vi "Exposure-Brickwall Noise.vi"(1 "seed":i32=-1, 7 "InvFilt Params":T3={"Min Frequency (Hz)"=0.0, "Max Frequency (Hz)"=0.0, "Length (points)"=301, "Sampling rate (Hz)"=0.0, "Delay (ms)"=301.0, "Linear phase"=FALSE}, 9 "Brickwall (T)":bool=TRUE, 11 "error in (no error)":errorcluster) -> (4 "Noise":dbl[](array[numeric]), 8 "dB":dbl[](array[numeric]), 15 "error out":errorcluster)   [LabVIEW 2020]
uses:
  epl-cal-vi-lib/Inverse Filter VIs/InvFilt-Params.ctl
  epl-vi-lib/Signal Synthesis VIs/Controls/Advanced Filter XCtl/Filter Data.ctl
  epl-vi-lib/Signal Synthesis VIs/Filter VIs/Filter-Bandwidth Units.ctl
  epl-vi-lib/Signal Synthesis VIs/Waveform VIs/Noise VIs/Noise-Globals.vi
  epl-vi-lib/Utility VIs/Math VIs/FFT x(t) to dB,Degrees (1D).vi
  epl-vi-lib/Utility VIs/Math VIs/Linear to dB (array).vi
  <vilib>/Analysis/NI_AALBase.lvlib
  epl-vi-lib/Signal Synthesis VIs/Controls/Advanced Filter XCtl/Advanced Filter XCtl.xctl
panel:
  in  "Filter in":T1={"Type"=enum."Bandpass", "CF (kHz)"=0.0, "BW (kHz)"=0.0, "Cascade"=TRUE, "Quadrature"=FALSE, "Scale Factor"=0.0, "Stages"=[], "Class"=enum."Elliptic", "Order"=7, "BWUnits"=enum."Linear"} {"Stages"."IIR Filter"."Forward Coefficients" format="%.4f"; "Stages"."IIR Filter"."Reverse Coefficients" format="%.4f"}
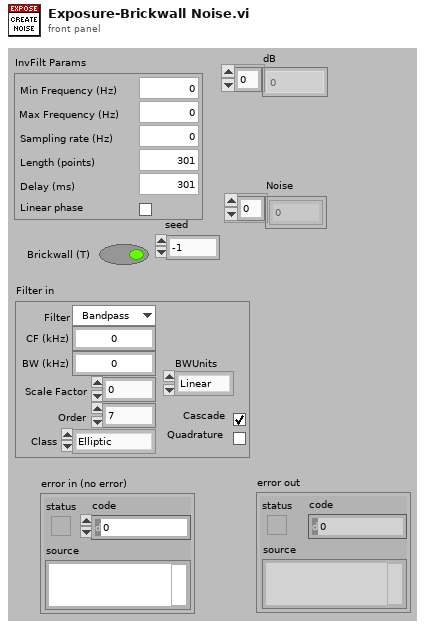
[diagram p1: front panel]
types:
  T1 = typedef "Advanced Filter XCtl.xctl/Filter Data.ctl" = cluster{"Type":enum16{"Lowpass", "Highpass", "Bandpass", "Bandstop", "OFF"}, "CF (kHz)":dbl, "BW (kHz)":dbl, "Cascade":bool, "Quadrature":bool, "Scale Factor":dbl, "Stages":cluster{"IIR Filter":cluster{"filter structure":enum32{"IIR 2nd Order", "IIR 4th Order"}, "Reverse Coefficients":dbl[], "Forward Coefficients":dbl[]}, "State":dbl[]}[], "Class":enum16{"Elliptic", "Butterworth"}, "Order":i32, "BWUnits":T2}
  T2 = typedef "Filter-Bandwidth Units.ctl" = enum16{"Linear", "Octaves", "Min-Max"}
  T3 = typedef "InvFilt-Params.ctl" = cluster{"Min Frequency (Hz)":dbl, "Max Frequency (Hz)":dbl, "Length (points)":i32, "Sampling rate (Hz)":dbl, "Delay (ms)":dbl, "Linear phase":bool}
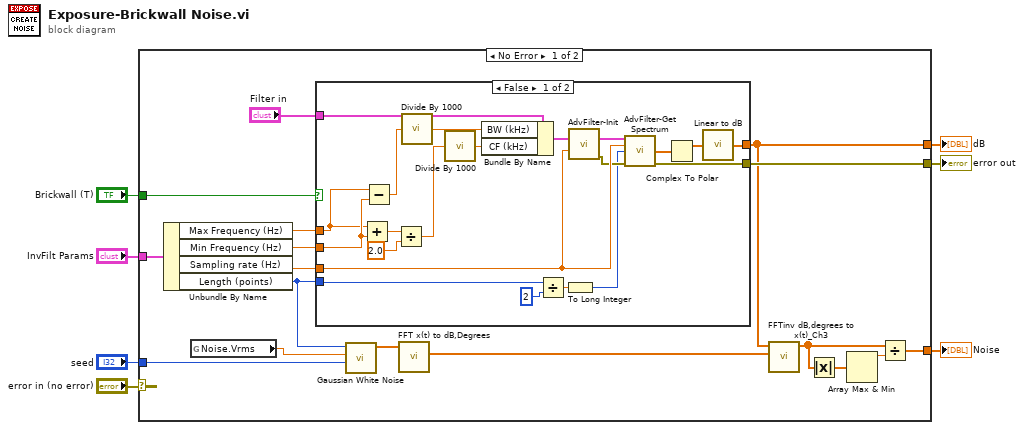
[diagram p0: block diagram]
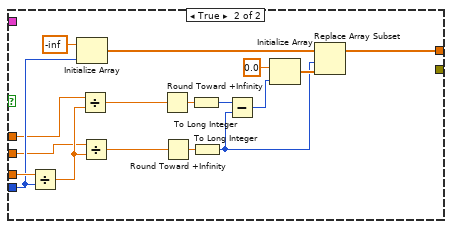
[diagram p2: hidden frame]
diagram:
  n1 = case shown="No Error" "error in (no error)" {
    selector: "error in (no error)" -> [_ w63]
    tunnel: [w11 w63] -> w6
    tunnel: "InvFilt Params" -> [w24 _]
    tunnel: [w18 _] -> w4
    tunnel: "Brickwall (T)" -> [w13 _]
    tunnel: [w10 _] -> w2
    tunnel: "seed" -> [w9 _]
    frame No Error {
      n2 = Unbundle By Name(w24) -> ("Max Frequency (Hz)"=w15:dbl, "Min Frequency (Hz)"=w14:dbl, "Sampling rate (Hz)"=w17:dbl, "Length (points)"=w16:i32)
      n3 = global read "Noise-Globals.vi" "Noise.Vrms"() -> (w8:dbl)
      n4 = case shown="False" w13 {
        tunnel: w17 -> [w36 w52]
        tunnel: w16 -> [w28 w51]
        tunnel: w15 -> [w40 w50]
        tunnel: w14 -> [w41 w49]
        tunnel: [w29 w46] -> w10
        tunnel: "Filter in" -> [w43 _]
        tunnel: [w34 _] -> w11
        frame False {
          n5 = Add(x=w40, y=w41) -> (x+y=w45:dbl)
          n6 = Subtract(x=w40, y=w41) -> (x-y=w39:dbl)
          n7 = Divide(x=w45, y=2.0) -> (x/y=w42:dbl)
          n8 = call "Divide By 1000.vi"("X"=w39) -> ("X/1000"=w33:dbl)
          n9 = call "Divide By 1000.vi"("X"=w42) -> ("X/1000"=w32:dbl)
          n10 = Bundle By Name(cluster=w43, "BW (kHz)"=w33, "CF (kHz)"=w32) -> (w38:T1)
          n11 = Divide(x=w28, y=2) -> (x/y=w26:dbl)
          n12 = To Long Integer(number=w26) -> (32bit integer=w25:i32)
          n13 = call "AdvFilter-Init.vi"("Filter"=w38, "Sampling rate (Hz)"=w36) -> ("Filter out"=w37:T1, "error out"=w35:errorcluster)  [unwired: 12 in]
          n14 = call "AdvFilter-Get Spectrum.vi"("Filter in"=w37, "Sampling Rate (Hz)"=w36, "Npts"=w25, "error in (no error)"=w35) -> ("spectrum"=w31:cdb[], "error out"=w34:errorcluster)  [unwired: 9 in, 1 out]
          n15 = Complex To Polar(r * e^(i*theta)=w31) -> (r=w30:dbl[])  [unwired: 1 out]
          n16 = call-poly "Linear to dB.vi"("linear"=w30) -> ("dB"=w29:dbl[])
        }
        frame True {
          n17 = Divide(x=w52, y=w51) -> (x/y=w59:dbl)
          n18 = Initialize Array(-inf ("element"), w51) -> (w47:dbl[])
          n19 = Divide(x=w50, y=w59) -> (x/y=w53:dbl)
          n20 = Divide(x=w49, y=w59) -> (x/y=w55:dbl)
          n21 = Round Toward +Infinity(x=w53) -> (ceil(x): smallest int >= x=w54:dbl)
          n22 = Round Toward +Infinity(x=w55) -> (ceil(x): smallest int >= x=w56:dbl)
          n23 = To Long Integer(number=w54) -> (32bit integer=w48:i32)
          n24 = To Long Integer(number=w56) -> (32bit integer=w57:i32)
          n25 = Subtract(x=w48, y=w57) -> (x-y=w58:i32)
          n26 = Initialize Array(0.0 ("element"), w58) -> (w61:dbl[])
          n27 = Replace Array Subset(array=w47, new element=w61, index=w57) -> (w46:dbl[])
        }
      }
      n28 = call <vilib>:"Gaussian White Noise.vi"("seed"=w9, "standard deviation"=w8, "samples"=w16) -> ("Gaussian noise pattern"=w19:dbl[])  [unwired: 7 in, 1 out]
      n29 = call-poly "FFT x(t) to dB,Degrees.vi"("X"=w19) -> ("+Freq Phase of FFT (degrees)"=w23:dbl[])  [unwired: 8 in, 2 out]
      n30 = call "FFTinv dB,degrees to x(t)_Ch3.vi"("+Freq Phase of FFT (degrees)"=w23, "+Freq. Mag of FFT (rms dB)"=w10) -> ("X(t)"=w20:dbl[])  [unwired: 8 in, 1 out]
      n31 = Absolute Value(x=w20) -> (abs(x)=w22:dbl[])
      n32 = Array Max & Min(array=w22) -> (max value=w21:dbl)  [unwired: 3 out]
      n33 = Divide(x=w20, y=w21) -> (x/y=w18:dbl[])
    }
    frame Error {
    }
  }
  "error out" <- w6
  "Noise" <- w4
  "dB" <- w2
